vi "CurrentSequenceStatus.vi"() -> ()   [LabVIEW 2018]
panel:
  out "Array":T1(array[cluster])
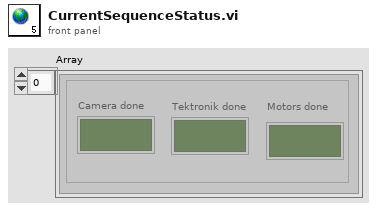
[diagram p1: front panel]
types:
  T1 = cluster{"Camera done":bool, "Tektronik done":bool, "Motors done":bool}[]
diagram:
